vi "draw_pointCollection.vi"(8 "error in (no error)":errorcluster, 10 "Display State In":T1={"current frame index"=0, "number of images"=0, "ROI (frames)"={"ROI"=[]}, "control refs"={"frame"=refnum, "image"=refnum, "saveROIsButton"=refnum, "loadImageSwitch"=refnum, "loadROIsSwitch"=refnum, "saveROIsSwitch"=refnum, "loadImagePath"=refnum, "loadROIPath"=refnum, "redraw"=refnum}, "calibration"={"x"=0.0, "y"=0.0, "x unit"=enum."um", "y unit"=enum."um"}, "xpaths"={"x offset"="", "y offset"="", "z offset"=""}, "offset"=refnum, "XML description"="", "number of ROIs"=0.0, "ROI Tool Buttons Visible"={"Zoom Tool"=TRUE, "Selection Tool"=TRUE, "Pan Tool"=TRUE, "Point Tool"=TRUE, "Line Tool"=TRUE, "Rectangle Tool"=TRUE, "Rotated Rectangle Tool"=TRUE, "Polyline Tool"=TRUE, "Polygon Tool"=TRUE, "Freehand Tool"=TRUE, "Closed Freehand Tool"=TRUE, "Ellipse Tool"=TRUE, "Annulus Tool"=TRUE}, "ROI color"=6618880, "enable ROI numbering?"=FALSE, "selected path to save ROIs"=path "", "starting path"=path "", "array of overlays"=[], "pointCollection"=refnum, "ROImode"=enum."none", "selected point ID"=1.0, "point radius"=0, "point colours"=[], "PlotAreaSize"={"Width"=0, "Height"=0}, "last action"=enum."not specified"} {"array of overlays"."overlay size" min=1}, 11 "ImageCollection in":refnum<class "ImageCollection.lvclass">) -> (0 "error out":errorcluster, 2 "Display State Out":T1={"current frame index"=0, "number of images"=0, "ROI (frames)"={"ROI"=[]}, "control refs"={"frame"=refnum, "image"=refnum, "saveROIsButton"=refnum, "loadImageSwitch"=refnum, "loadROIsSwitch"=refnum, "saveROIsSwitch"=refnum, "loadImagePath"=refnum, "loadROIPath"=refnum, "redraw"=refnum}, "calibration"={"x"=0.0, "y"=0.0, "x unit"=enum."um", "y unit"=enum."um"}, "xpaths"={"x offset"="", "y offset"="", "z offset"=""}, "offset"=refnum, "XML description"="", "number of ROIs"=0.0, "ROI Tool Buttons Visible"={"Zoom Tool"=TRUE, "Selection Tool"=TRUE, "Pan Tool"=TRUE, "Point Tool"=TRUE, "Line Tool"=TRUE, "Rectangle Tool"=TRUE, "Rotated Rectangle Tool"=TRUE, "Polyline Tool"=TRUE, "Polygon Tool"=TRUE, "Freehand Tool"=TRUE, "Closed Freehand Tool"=TRUE, "Ellipse Tool"=TRUE, "Annulus Tool"=TRUE}, "ROI color"=6618880, "enable ROI numbering?"=FALSE, "selected path to save ROIs"=path "", "starting path"=path "", "array of overlays"=[], "pointCollection"=refnum, "ROImode"=enum."none", "selected point ID"=1.0, "point radius"=0, "point colours"=[], "PlotAreaSize"={"Width"=0, "Height"=0}, "last action"=enum."not specified"} caption="State" {"array of overlays"."overlay size" min=1}, 3 "ImageCollection out":refnum<class "ImageCollection.lvclass">)   [LabVIEW 2010, in "XImage.xctl"]
uses:
  XImage.xctl
  state.ctl
  classes/SpaceVector/SpaceVector/SpaceVector.lvclass
  classes/PointCollection/PointCollection/PointCollection.lvclass
  ROI_frames_cluster.ctl
  control_refs_cluster.ctl
  calibration_cluster.ctl
  enumerations/unit.ctl
  xpath_cluster.ctl
  overlays_cluster.ctl
  ROI_mode_enum.ctl
  last_action_enum.ctl
  classes/ImageCollection/ImageCollection/ImageCollection.lvclass
  classes/ImageCollection/ImageCollection/add_mode_enum.ctl
  classes/PointCollection/PointCollection/mode_enum.ctl
  classes/Image/Image/Image.lvclass
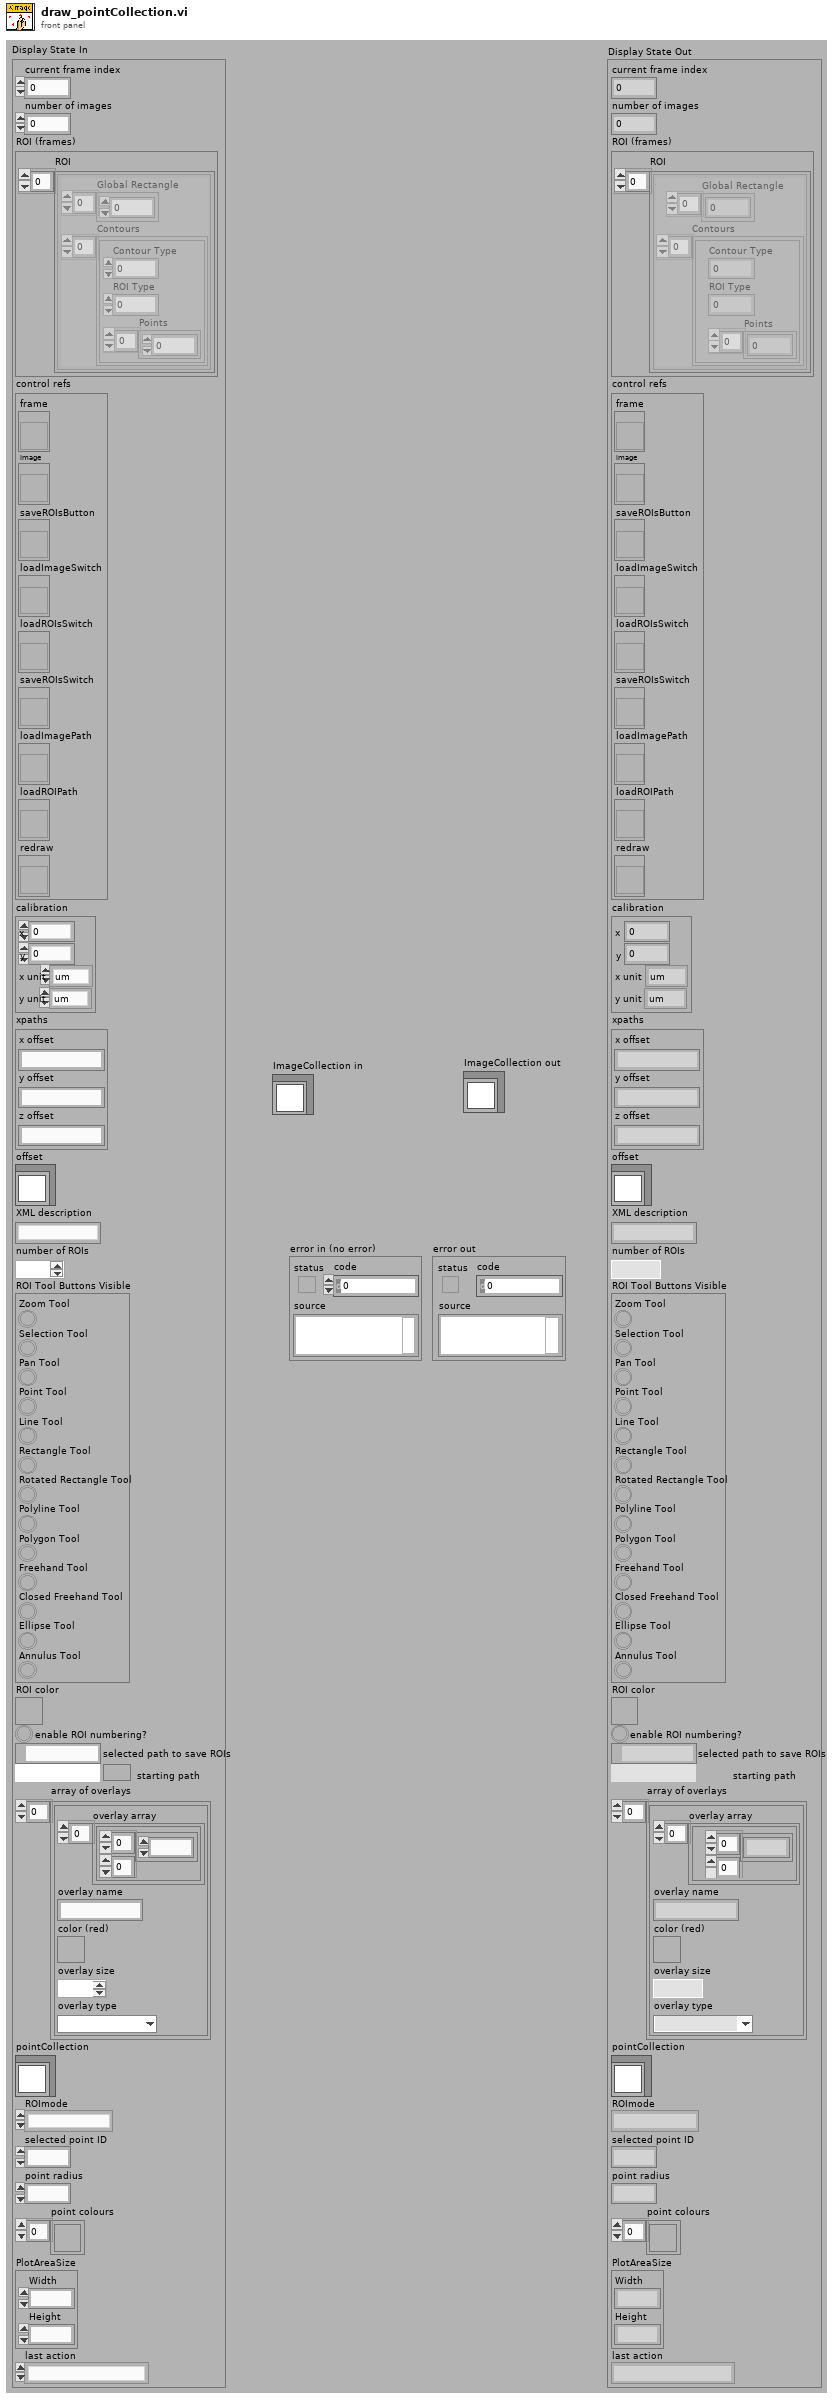
[diagram p1: front panel]
types:
  T1 = typedef "XImage.xctl/state.ctl" = cluster{"current frame index":i32, "number of images":i32, "ROI (frames)":T2, "control refs":T3, "calibration":T4, "xpaths":T6, "offset":refnum<class "SpaceVector.lvclass">, "XML description":string, "number of ROIs":dbl, "ROI Tool Buttons Visible":cluster{"Zoom Tool":bool, "Selection Tool":bool, "Pan Tool":bool, "Point Tool":bool, "Line Tool":bool, "Rectangle Tool":bool, "Rotated Rectangle Tool":bool, "Polyline Tool":bool, "Polygon Tool":bool, "Freehand Tool":bool, "Closed Freehand Tool":bool, "Ellipse Tool":bool, "Annulus Tool":bool}, "ROI color":u32, "enable ROI numbering?":bool, "selected path to save ROIs":path, "starting path":path, "array of overlays":T7[], "pointCollection":refnum<class "PointCollection.lvclass">, "ROImode":T8, "selected point ID":dbl, "point radius":i32, "point colours":u32[], "PlotAreaSize":cluster{"Width":u32, "Height":u32}, "last action":T9}
  T2 = typedef "XImage.xctl/ROI_frames_cluster.ctl" = cluster{"ROI":cluster{"Global Rectangle":i32[], "Contours":cluster{"Contour Type":u32, "ROI Type":u32, "Points":i32[]}[]}[]}
  T3 = typedef "XImage.xctl/control_refs_cluster.ctl" = cluster{"frame":refnum<vi>, "image":refnum<vi>, "saveROIsButton":refnum<vi>, "loadImageSwitch":refnum<vi>, "loadROIsSwitch":refnum<vi>, "saveROIsSwitch":refnum<vi>, "loadImagePath":refnum<vi>, "loadROIPath":refnum<vi>, "redraw":refnum<vi>}
  T4 = typedef "XImage.xctl/calibration_cluster.ctl" = cluster{"x":dbl, "y":dbl, "x unit":T5, "y unit":T5}
  T5 = typedef "Image.lvclass/unit.ctl" = enum16{"um", "s"}
  T6 = typedef "XImage.xctl/xpath_cluster.ctl" = cluster{"x offset":string, "y offset":string, "z offset":string}
  T7 = typedef "XImage.xctl/overlays_cluster.ctl" = cluster{"overlay array":cluster{i32[][]}[], "overlay name":string, "color (red)":u32, "overlay size":i32, "overlay type":enum16{"crosshair", "circle"}}
  T8 = typedef "XImage.xctl/ROI_mode_enum.ctl" = enum16{"none", "IMAQROIs", "PointCollection"}
  T9 = typedef "XImage.xctl/last_action_enum.ctl" = enum16{"not specified", "image loaded", "frame changed", "ROIs changed"}
  T10 = typedef "ImageCollection.lvclass/add_mode_enum.ctl" = enum16{"instance", "copy"}
  T11 = typedef "PointCollection.lvclass/mode_enum.ctl" = enum16{"points first", "dimensions first"}
  T12 = cluster{"Left":i32, "Top":i32, "Right":i32, "Bottom":i32}
  T13 = typedef "IMAQ Image.ctl" = refnum<image>
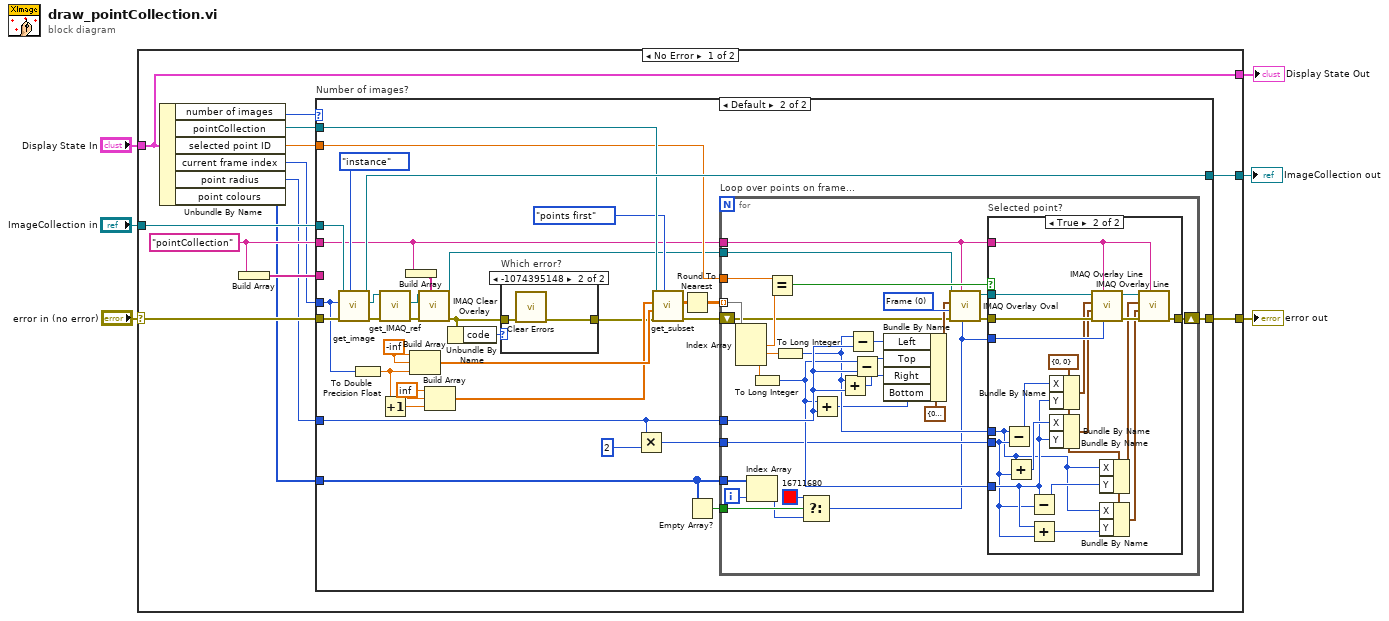
[diagram p0: block diagram]
diagram:
  n1 = case shown="No Error" "error in (no error)" {
    selector: "error in (no error)" -> [w9 w109]
    tunnel: [w18 w109] -> w1
    tunnel: "Display State In" -> [w10 w107]
    tunnel: "ImageCollection in" -> [w17 w108]
    tunnel: [w16 w108] -> w3
    tunnel: [w10 w107] -> w2
    frame No Error {
      w19 = "pointCollection" ("Group")
      n2 = Unbundle By Name(w10) -> ("number of images"=w14:i32, "pointCollection"=w12:refnum<class "PointCollection.lvclass">, "selected point ID"=w11:dbl, "current frame index"=w13:i32, "point radius"=w8:i32, "point colours"=w7:u32[])
      n3 = Build Array(w19) -> (w15:string[])
      n4 = case "Number of images?" shown="Default" w14 {
        tunnel: w19 -> [_ w22]
        tunnel: [w21 w54] -> w18
        tunnel: w17 -> [w20 w53]
        tunnel: [w20 w52] -> w16
        tunnel: w12 -> [_ w51]
        tunnel: w15 -> [_ _]
        tunnel: w9 -> [w21 w50]
        tunnel: w13 -> [_ w37]
        tunnel: w8 -> [_ w33]
        tunnel: w11 -> [_ w35]
        tunnel: w7 -> [_ w29]
        frame 0 {
        }
        frame Default {
          w44 = inf
          w45 = -inf
          n5 = call-dynamic "get_image.vi"("get image as..."=add_mode_enum."instance", "error in (no error)"=w50, "index"=w37, "ImageCollection in"=w53) -> ("error out"=w48:errorcluster, "Image.lvclass"=w47:refnum<class "Image.lvclass">, "ImageCollection out"=w52:refnum<class "ImageCollection.lvclass">)  [unwired: 5 in]
          n6 = To Double Precision Float(number=w37) -> (double precision float=w43:dbl)
          n7 = call-dynamic "get_IMAQ_ref.vi"("error in (no error)"=w48, "Image.lvclass in"=w47) -> ("error out"=w27:errorcluster, "Image"=w25:T13)  [unwired: 5 in, 3 out]
          n8 = Increment(x=w43) -> (x+1=w42:dbl)
          n9 = Build Array(w22) -> (w23:string[])
          n10 = Build Array(w45, w45, w43) -> (w39:dbl[])
          n11 = call "IMAQ Clear Overlay"("Groups"=w23, "error in (no error)"=w27, "Image"=w25) -> ("error out"=w26:errorcluster, "Image Out"=w24:T13)  [unwired: 7 in]
          n12 = Build Array(w44, w44, w42) -> (w38:dbl[])
          n13 = Unbundle By Name(w26) -> ("code"=w40:i32)
          n14 = case "Which error?" shown="-1074395148" w40 {
            tunnel: w26 -> [w55 w57]
            tunnel: [w55 w56] -> w30
            frame Default {
            }
            frame -1074395148 {
              n15 = call <vilib>:"Clear Errors.vi"("error in (no error)"=w57) -> ("error out"=w56:errorcluster)  [unwired: 6 in]
            }
          }
          n16 = Multiply(x=w33, y=2) -> (x*y=w31:i32)
          n17 = call "get_subset.vi"("retrieval mode"=mode_enum."points first", "error in (no error)"=w30, "min (x/y/z)"=w39, "max (x/y/z)"=w38, "PointCollection in"=w51) -> ("error out"=w49:errorcluster, "points"=w36:dbl[][])  [unwired: 4 in, 1 out]
          n18 = Round To Nearest(number=w36) -> (nearest integer value=w34:dbl[][])
          n19 = Empty Array?(array=w29) -> (empty?=w28:bool)
          n20 = for "Loop over points on frame..." {
            shift-right: [w76] -> w54
            shift-left: w49 -> [w62]
            tunnel: w34 -> [w84] mode=indexing
            tunnel: w24 -> [w63]
            tunnel: w33 -> [w72]
            tunnel: w22 -> [w61]
            tunnel: w35 -> [w81]
            tunnel: w31 -> [w69]
            tunnel: w29 -> [w67]
            tunnel: w28 -> [w66]
            i -> [w68]
            w86 = u32 0 items=["Frame", "Fill"] ("Drawing Mode (Frame)")
            n21 = Index Array(array=w84) -> (element #1=w80:dbl, element #2=w78:dbl, element #3=w79:dbl)  [unwired: 3 in]
            n22 = Index Array(array=w67, index=w68) -> (element=w64:u32)
            n23 = To Long Integer(number=w79) -> (32bit integer=w71:i32)
            n24 = Equal?(x=w81, y=w80) -> (x = y?=w74:bool)
            n25 = To Long Integer(number=w78) -> (32bit integer=w70:i32)
            n26 = Select(t=u32 16711680 ("Color"), s=w66, f=w64) -> (s? t:f=w58:u32)
            n27 = Add(x=w71, y=w72) -> (x+y=w59:i32)
            n28 = Add(x=w70, y=w72) -> (x+y=w60:i32)
            n29 = Subtract(x=w70, y=w72) -> (x-y=w73:i32)
            n30 = Subtract(x=w71, y=w72) -> (x-y=w83:i32)
            n31 = Bundle By Name(cluster=T12 {"Left"=0, "Top"=0, "Right"=0, "Bottom"=0} ("Bounding Rectangle"), "Left"=w73, "Top"=w83, "Right"=w60, "Bottom"=w59) -> (w82:T12)
            n32 = call "IMAQ Overlay Oval"("Color"=w58, "Group"=w61, "error in (no error)"=w62, "Drawing Mode (Frame)"=w86, "Bounding Rectangle"=w82, "Image"=w63) -> ("error out"=w77:errorcluster, "Image Out"=w75:T13)  [unwired: 4 in]
            n33 = case "Selected point?" shown="True" w74 {
              tunnel: w77 -> [w87 w106]
              tunnel: w58 -> [_ w105]
              tunnel: [w87 w102] -> w76
              tunnel: w75 -> [_ w101]
              tunnel: w61 -> [_ w100]
              tunnel: w71 -> [_ w92]
              tunnel: w70 -> [_ w88]
              tunnel: w69 -> [_ w91]
              frame False {
              }
              frame True {
                w95 = cluster{"X":i32, "Y":i32} {"X"=0, "Y"=0} ("Start Point")
                n34 = Subtract(x=w88, y=w91) -> (x-y=w94:i32)
                n35 = Add(x=w88, y=w91) -> (x+y=w93:i32)
                n36 = Subtract(x=w92, y=w91) -> (x-y=w90:i32)
                n37 = Add(x=w92, y=w91) -> (x+y=w89:i32)
                n38 = Bundle By Name(cluster=w95, "X"=w94, "Y"=w92) -> (w99:cluster{"X":i32, "Y":i32})
                n39 = Bundle By Name(cluster=w95, "X"=w93, "Y"=w92) -> (w98:cluster{"X":i32, "Y":i32})
                n40 = call "IMAQ Overlay Line"("Color"=w105, "Group"=w100, "error in (no error)"=w106, "End Point"=w98, "Start Point"=w99, "Image"=w101) -> ("error out"=w103:errorcluster, "Image Out"=w104:T13)  [unwired: 4 in]
                n41 = Bundle By Name(cluster=w95, "X"=w88, "Y"=w90) -> (w97:cluster{"X":i32, "Y":i32})
                n42 = Bundle By Name(cluster=w95, "X"=w88, "Y"=w89) -> (w96:cluster{"X":i32, "Y":i32})
                n43 = call "IMAQ Overlay Line"("Group"=w100, "error in (no error)"=w103, "End Point"=w96, "Start Point"=w97, "Image"=w104) -> ("error out"=w102:errorcluster)  [unwired: 5 in, 1 out]
              }
            }
          }
        }
      }
    }
    frame Error {
    }
  }
  "Display State Out" <- w2
  "ImageCollection out" <- w3
  "error out" <- w1
